vi "SDT_GenerateBHFileBlockHeaderDecayFCSMCS.vi"(7 "ModuleNo":u32, 10 "ArrayLengths":i32[](array[numeric]), 11 "data_block_offs":i32) -> (2 "BHFileBlockHeaders":T1[](array[typedef]), 3 "BlockHeaderLength":i32)   [LabVIEW 2017]
doc: "This VI is a SubVI to SDT_WriteFile.vi. It populates the clusters BHFileBlockHeader ready to be written to file. \nFor a description of the *.sdt file format see: SPC_data_file_structure.h\n\ninfo@becker-hickl.com"
uses:
  SPC_Wrappers/SPC_Controls/BHFileBlockHeader.ctl
  SPC_Wrappers/SPC_Controls/BlockType_Contents.ctl
  SPC_Wrappers/SPC_Controls/BlockType_DataType.ctl
  SPC_Wrappers/SPC_Controls/BlockType_CreationMode.ctl
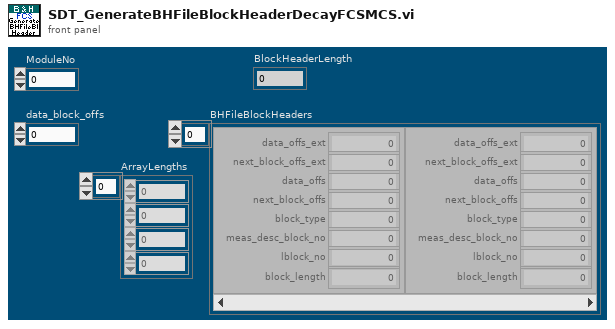
[diagram p1: front panel]
types:
  T1 = typedef "BHFileBlockHeader.ctl" = cluster{"data_offs_ext":u8, "next_block_offs_ext":u8, "data_offs":u32, "next_block_offs":u32, "block_type":u16, "meas_desc_block_no":i16, "lblock_no":u32, "block_length":u32}
  T2 = typedef "BlockType_DataType.ctl" = u16
  T3 = typedef "BlockType_Contents.ctl" = u16
  T4 = enum16{"big-endian, network order", "native, host order", "little-endian"}
  T5 = typedef "BlockType_CreationMode.ctl" = u16
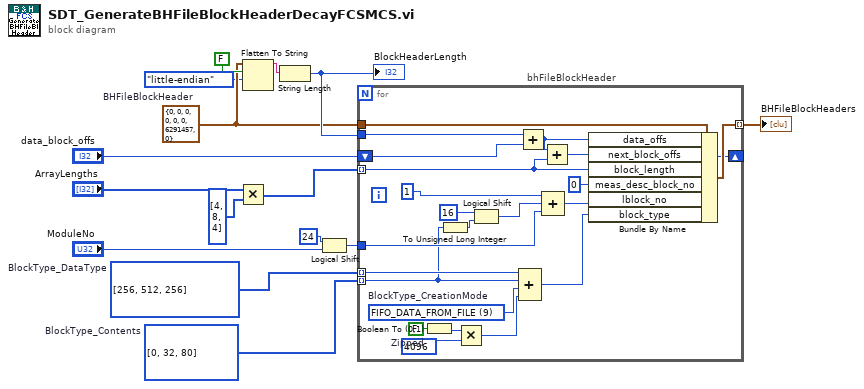
[diagram p0: block diagram]
diagram:
  w7 = T1 {"data_offs_ext"=0, "next_block_offs_ext"=0, "data_offs"=0, "next_block_offs"=0, "block_type"=0, "meas_desc_block_no"=0, "lblock_no"=6291457, "block_length"=0}  # BHFileBlockHeader
  w4 = T2[] [256, 512, 256] items=["DATA_USHORT (U16)"=0, "DATA_ULONG (U32)"=256, "DATA_DBL (DBL64)"=512]  # BlockType_DataType
  w3 = T3[] [0, 32, 80] items=["DECAY_BLOCK"=0, "PAGE_BLOCK"=16, "FCS_BLOCK"=32, "FIDA_BLOCK"=48, "FILDA_BLOCK"=64, "MCS_BLOCK"=80, "IMG_BLOCK"=96, "MCST_BLOCK"=112, "IMG_MCS_BLOCK"=128, "MOM_BLOCK"=144, "IMG_INT_BLOCK"=160, "IMG_WF_BLOCK"=176, "IMG_LIFE_BLOCK"=192]  # BlockType_Contents
  n1 = Multiply(x="ArrayLengths", y=i32[] [4, 8, 4]) -> (x*y=w2:i32[])
  n2 = Flatten To String(anything=w7, prepend array or string size? (T)=FALSE, byte order (0:big-endian, network order)=T4."little-endian") -> (data string=w5:string)  [unwired: 1 in, 2 out]
  n3 = String Length(string=w5) -> (length=w9:i32)
  "BlockHeaderLength" <- w9
  n4 = Logical Shift(y=i16 24, x="ModuleNo") -> (x << y=w11:u32)
  n5 = for "bhFileBlockHeader" {
    tunnel: w9 -> [w35]
    tunnel: w4 -> [w22] mode=indexing
    tunnel: w3 -> [w21] mode=indexing
    tunnel: w7 -> [w36]
    tunnel: [w37] -> w13 mode=indexing
    tunnel: w2 -> [w18] mode=indexing
    shift-right: [w28] -> _
    shift-left: "data_block_offs" -> [w27]
    tunnel: w11 -> [w23]
    w33 = FALSE  # Zipped
    w34 = T5 9 items=["NOT_USED"=0, "MEAS_DATA"=1, "FLOW_DATA"=2, "MEAS_DATA_FROM_FILE"=3, "CALC_DATA"=4, "SIM_DATA"=5, "FIFO_DATA"=8, "FIFO_DATA_FROM_FILE"=9, "MOM_DATA"=10, "MOM_DATA_FROM_FILE"=11]  # BlockType_CreationMode
    n6 = Boolean To (0,1)(Boolean=w33) -> (0, 1=w32:i16)
    n7 = To Unsigned Long Integer(number=w21) -> (unsigned 32bit integer=w20:u32)
    n8 = Multiply(x=w32, y=u16 4096) -> (x*y=w30:u16)
    n9 = Logical Shift(y=u16 16, x=w20) -> (x << y=w26:u32)
    n10 = Add(x=w35, y=w27) -> (x+y=w29:i32)
    n11 = Compound Arithmetic op=ADD(w22, w21, w34, w30) -> (w19:T2)
    n12 = Add(x=w29, y=w18) -> (x+y=w28:i32)
    n13 = Compound Arithmetic op=ADD(1, w26, w23) -> (w25:u32)
    n14 = Bundle By Name(cluster=w36, "data_offs"=w29, "next_block_offs"=w28, "block_length"=w18, "meas_desc_block_no"=0, "lblock_no"=w25, "block_type"=w19) -> (w37:T1)
  }
  "BHFileBlockHeaders" <- w13
